vi "Dashboard Main.vi"() -> ()   [LabVIEW 2013]
uses:
  <vilib>/event_ctls.llb/eventvkey.ctl
  <vilib>/Rock Robotics/WPI/Dashboard/WPI_DashboardLogging Global.vi
  <vilib>/Utility/config.llb/Write Key (String).vi
  <vilib>/Utility/config.llb/Write Key (I32).vi
  <vilib>/Utility/config.llb/NI_LVConfig.lvlib
panel:
  out "code":string
  out "Image Message":string="Timeout in Camera Communications"
  in  "Rec Mode":enum32{"Stop", "Record", "Playback"}(radio)
  in  "Dashboard Tab":T1(tab)
  in  "Camera Settings":T2={"Frame Rate"=30, "Compression"=30, "Size"=1} {"Frame Rate" scale=1.0..30.0; "Size" items=["640x480", "320x240", "160x120"]}
  out "MotorSliders R":cluster{"MotorSlide1":dbl, "MotorSlide2":dbl} {"MotorSlide2" scale=-1.0..1.0 scale format="%#_2e"; "MotorSlide1" scale=-1.0..1.0 scale format="%#_2e"}
  out "MotorChart R":cluster{"Numeric":dbl, "Numeric":dbl}(graph)
  out "MotorSliders L":T3 {"MotorSlide4 2" scale=0.0..14.0 scale format="%#_2e"; "MotorSlide2" scale=-1.0..1.0 scale format="%#_2e"; "MotorSlide1" scale=-1.0..1.0 scale format="%#_2e"}
  out "MotorChart L":T4(graph)
  out "JS1 Z":dbl(slide) scale=-1.0..1.0 scale format="%#_2e"
  out "Joystick 1":cluster{"X":dbl, "Y":dbl}[](graph)
  out "JS Buttons 1":T5
  out "JS2 Z":dbl(slide) scale=-1.0..1.0 scale format="%#_2e"
  out "Joystick 2":cluster{"X":dbl, "Y":dbl}[](graph)
  out "JS Buttons 2":T5
  out "Mode":T6(ring)=enum."Auto Disabled"
  out "Camera IP":string
  in  "DB Camera Config":bool
  out "fps":dbl format="%#.1g"
  out "Mbps":dbl format="%#.1g"
  out "Mbps 2":bool
  out "LED 1":bool
  in  "loadCode":bool
  in  "pick auto":string
  out "left":dbl
  out "right":dbl
  out "Waveform Chart":dbl[][](graph)
  in  "Checkbox 2":bool
  in  "Checkbox 1":bool
  in  "Test Slider":dbl(slide) scale=0.0..100.0 scale format="%#_3g"
  in  "On/Off":bool caption="Solenoid"
  in  "Test Name":u16(ring) items=["Select the test to run...", "Example Test", "-------------------------------", "List of tests is built in robot code.", "Replace with your own automated tests."]
  in  "Test Tree":string(tree)
  in  "Motor":cluster{"Value":dbl, "Enable":bool} {"Value" scale=-1.0..1.0 scale format="%#_3g"}
  out "Progress":T7 {"Test Progress" scale=0.0..100.0}
  in  "Rev/Fwd":cluster{"Forward":bool, "Reverse":bool}
  in  "Test Ring":u16(ring) items=["Auto", "Fixed indoor", "Fixed outdoor 1", "Fixed outdoor 2", "Fixed fluorescent 1", "Fixed fluorescent 2", "Hold current"]
  in  "Listbox":i32(listbox)
  out "Tree":string(tree)
  out "Camera Image":T8(plugin-control)
  in  "Enable":bool
  # "Left"
  # "Front"
  # "Right"
  # "Battery"
  # "This tab is a great place for autonomous settings and validation.\nCustomize by placing controls and indicators here and name to\nmatch Dashboard Variables on robot."
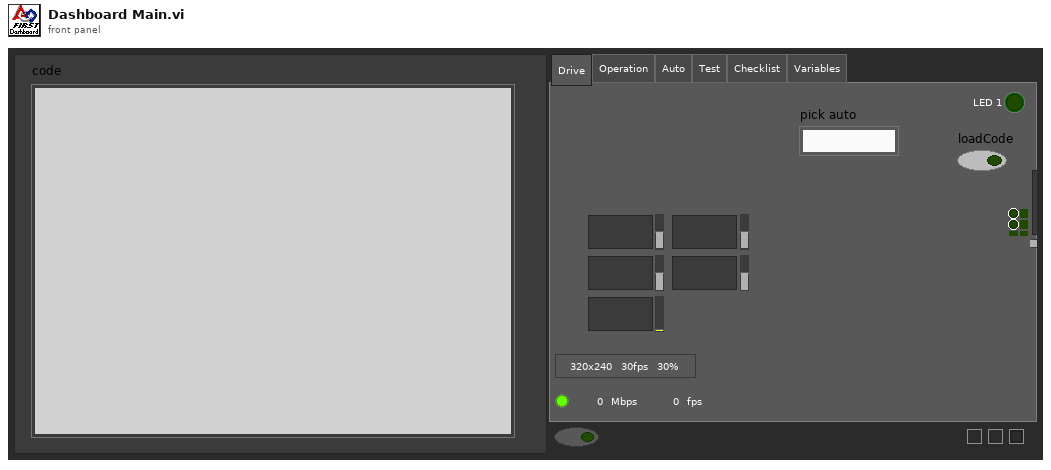
[diagram p1: front panel]
types:
  T1 = enum32{"Drive", "Operation", "Auto", "Test", "Checklist", "Variables"}
  T2 = cluster{"Frame Rate":i32, "Compression":i32, "Size":u16}
  T3 = cluster{"MotorSlide1":dbl, "MotorSlide2":dbl, "MotorSlide4 2":dbl}
  T4 = cluster{"Numeric":dbl, "Numeric":dbl, "Battery":sgl}
  T5 = cluster{bool, bool, bool, bool, bool, bool, bool, bool, bool, bool, bool, bool}
  T6 = enum8{"Tele-Op Disabled", "Tele-Op Enabled", "Auto Disabled", "Auto Enabled", "Test Disabled", "Test Enabled", ""}
  T7 = cluster{"Test Progress":u8, "Test Progress Text":string}
  T8 = typedef "IMAQ Image.ctl" = refnum<image>
  T9 = typedef "Image Type" = u32
  T10 = cluster{"Digital Inputs":bool[], "Digital Outputs":bool[]}
  T11 = cluster{"Competition mode":bool, "Robot Link":bool, "Autonomous":bool, "Enabled":bool, "E-Stop":bool, "Simulated":bool, "TestMode":bool, "Docked Window":bool}
  T12 = cluster{"Boolean Array[0]":bool, "Boolean Array[1]":bool, "Boolean Array[2]":bool, "Boolean Array[3]":bool, "Boolean Array[4]":bool, "Boolean Array[5]":bool, "Boolean Array[6]":bool, "Boolean Array[7]":bool, "Boolean Array[8]":bool, "Boolean Array[9]":bool, "Boolean Array[10]":bool, "Boolean Array[11]":bool}
  T13 = typedef "NI_LVConfig.lvlib/Config Data RefNum.ctl" = refnum<k1>
  T14 = typedef "eventvkey.ctl" = enum16{"ASCII", "Enter", "Return", "Shift", "Ctrl", "Alt", "Cmd", "Opt", "Caps", "NumLock", "Clear", "Break", "Up", "Down", "Left", "Right", "Insert", "Delete", "Home", "End", "PageUp", "PageDown", "Escape", "Help", "Pause", "ScrollLock", "F1", "F2", "F3", "F4", "F5", "F6", "F7", "F8", "F9", "F10", "F11", "F12", "F13", "F14", "F15", "F16", "F17", "F18", "F19", "F20", "F21", "F22", "F23", "F24", "Play", "VolumeUp", "VolumeDown", "Mute", "Two Byte Char"}
  T15 = cluster{"Image Size":bool, "Image Type":bool, "Pixel Value":bool, "ROI Information":bool, "Zoom Factor":bool}
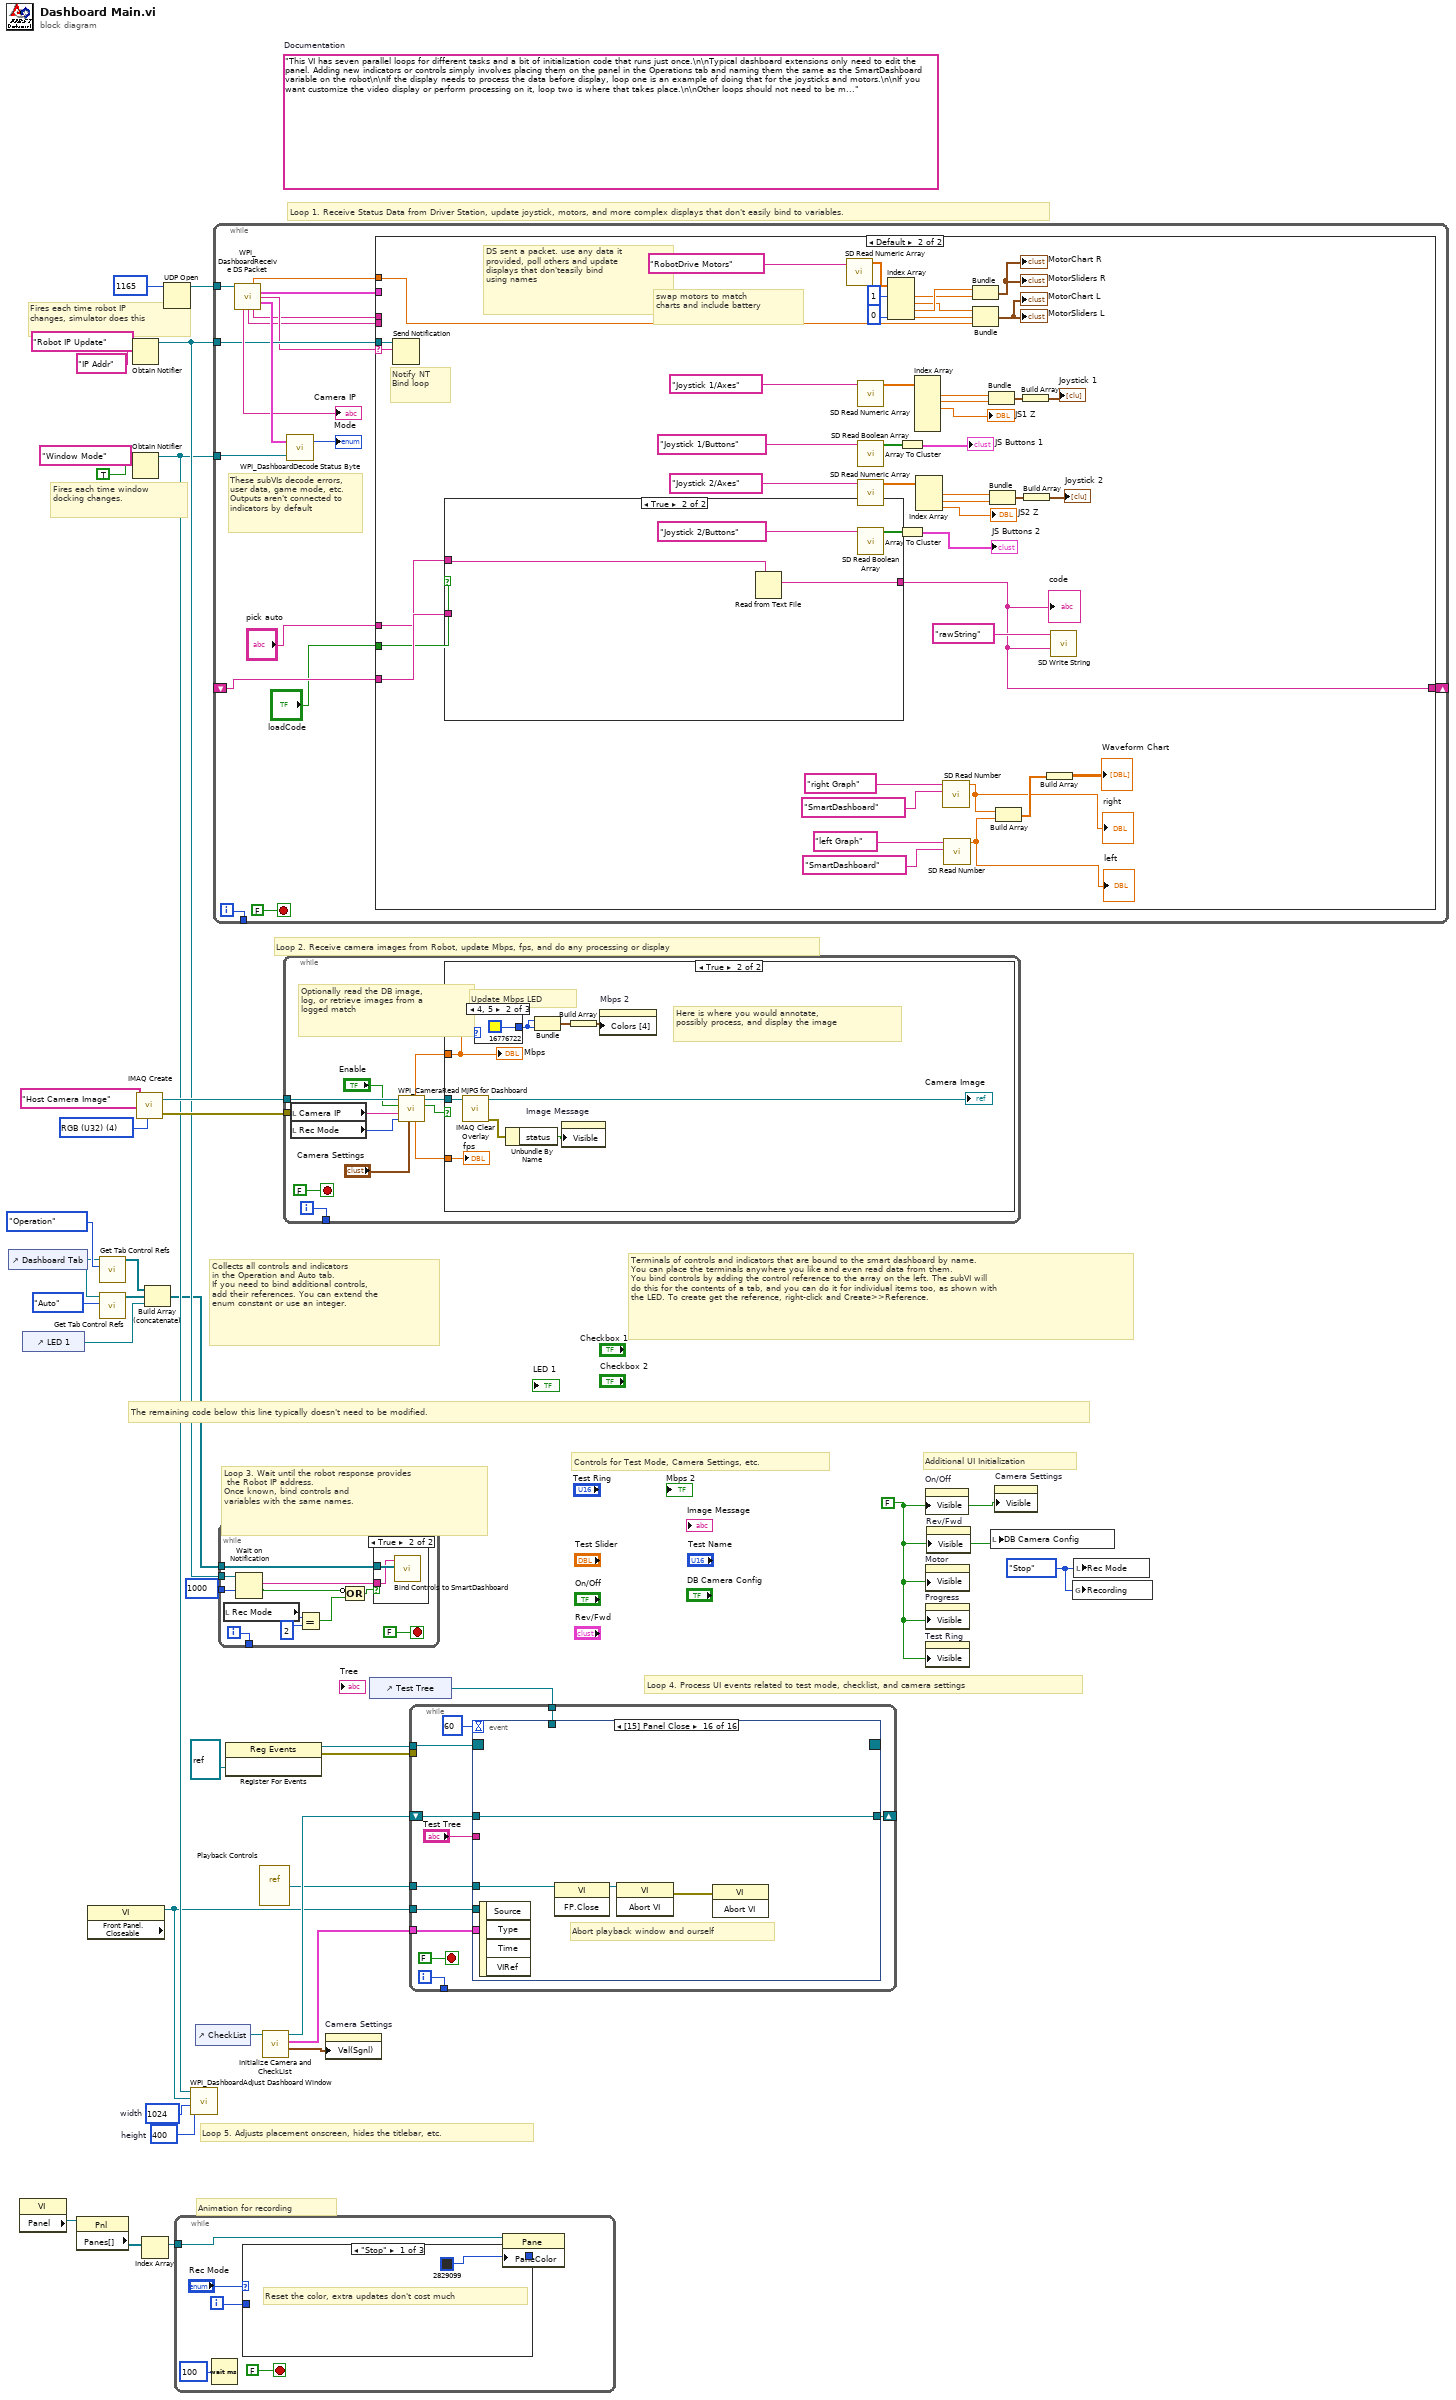
[diagram p0: block diagram]
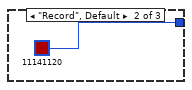
[diagram p2: hidden frame]
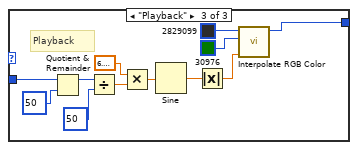
[diagram p3: hidden frame]
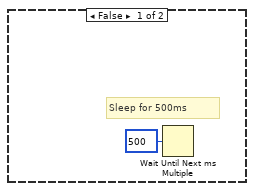
[diagram p5: hidden frame]
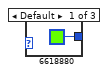
[diagram p6: hidden frame]
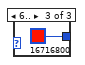
[diagram p7: hidden frame]
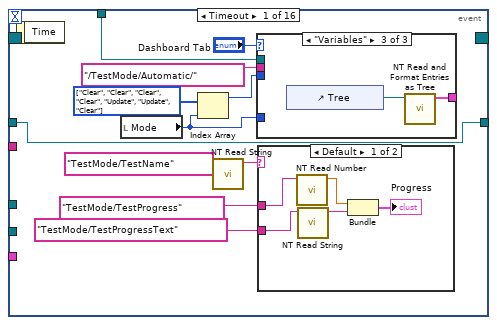
[diagram p8: hidden frame]
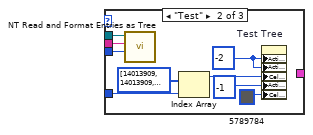
[diagram p10: hidden frame]
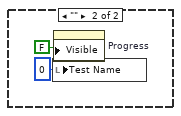
[diagram p11: hidden frame]
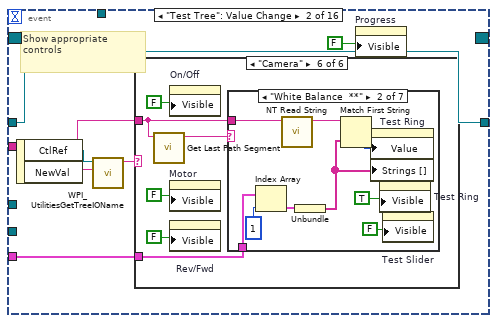
[diagram p12: hidden frame]
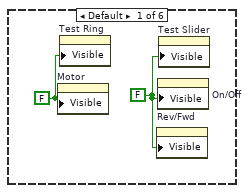
[diagram p13: hidden frame]
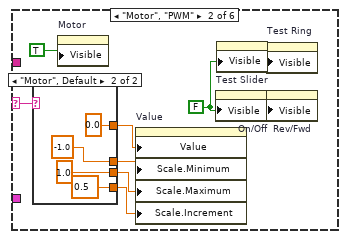
[diagram p14: hidden frame]
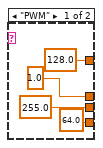
[diagram p15: hidden frame]
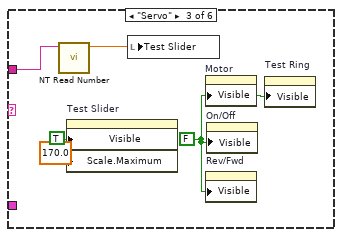
[diagram p16: hidden frame]
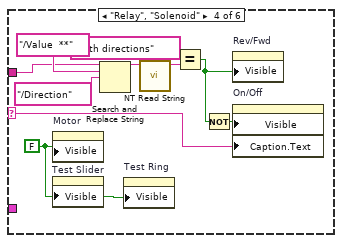
[diagram p17: hidden frame]
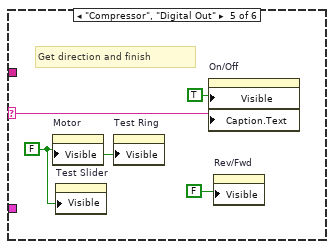
[diagram p18: hidden frame]
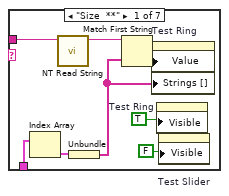
[diagram p19: hidden frame]
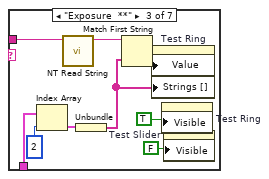
[diagram p20: hidden frame]
diagram:
  w8 = enum32{"Stop", "Record", "Playback"}."Stop" ("Rec Mode")
  w11 = 400  # height
  w12 = 1024  # width
  w25 = FALSE ("Visible")
  (unwired) "This VI has seven parallel loops for different tasks and a bit of initialization code that runs just once.\n\nTypical dashboard extensions only need to edit the panel. Adding new indicators or controls simply involves placing them on the panel in the Operations tab and naming them the same as the SmartDashboard variable on the robot\n\nIf the display needs to process the data before display, loop one is an example of doing that for the joysticks and motors.\n\nIf you want customize the video display or perform processing on it, loop two is where that takes place.\n\nOther loops should not need to be modified. They are pretty standard, and document the task they perform."  # Documentation
  w35 = T9 4 items=["Grayscale (U8)", "Grayscale (I16)", "Grayscale (SGL)", "Complex (CSG)", "RGB (U32)", "HSL (U32)", "RGB (U64)"] ("Image Type")
  # "Controls for Test Mode, Camera Settings, etc."
  # "Additional UI Initialization"
  # "Animation for recording"
  # "Fires each time robot IP\nchanges, simulator does this"
  # "Fires each time window\ndocking changes."
  # "Collects all controls and indicators\nin the Operation and Auto tab.\nIf you need to bind additional controls,\nadd their references. You can extend the\nenum constant or use an integer."
  # "The remaining code below this line typically doesn't need to be modified."
  # "Loop 4. Process UI events related to test mode, checklist, and camera settings"
  # "Terminals of controls and indicators that are bound to the smart dashboard by name.\nYou can place the terminals anywhere you like and even read data from them.\nYou bind controls by adding the control reference to the array on the left. The subVI will\ndo this for the contents of a tab, and you can do it for individual items too, as shown with\nthe LED. To create get the reference, right-click and Create>>Reference."
  # "Loop 3. Wait until the robot response provides\n the Robot IP address.\nOnce known, bind controls and\nvariables with the same names."
  # "Loop 5. Adjusts placement onscreen, hides the titlebar, etc."
  # "Loop 1. Receive Status Data from Driver Station, update joystick, motors, and more complex displays that don't easily bind to variables."
  # "Loop 2. Receive camera images from Robot, update Mbps, fps, and do any processing or display"
  n1 = control-ref of="Dashboard Tab"() -> (w6:refnum<vi>)
  n2 = property class="VI"() -> ("Panel"=w19:refnum<vi>)  [unwired: 2 in, 2 out]
  n3 = control-ref of="LED 1"() -> (w1:refnum<vi>)
  n4 = property class="Pnl"(reference=w19) -> ("Panes[]"=w20:refnum<vi>[])  [unwired: 1 in, 2 out]
  n5 = property class="VI" props=["Front Panel.Closeable"]() -> (reference out=w7:refnum<vi>)  [unwired: 2 in, 2 out]
  n6 = call <vilib>:"Get Tab Control Refs.vi"("Page Index"=T1."Operation" ("Dashboard Tab"), "TabControl in"=w6) -> ("ControlsOnPage"=w4:refnum<vi>[])  [unwired: 9 in]
  n7 = call <vilib>:"Get Tab Control Refs.vi"("Page Index"=T1."Auto" ("Dashboard Tab"), "TabControl in"=w6) -> ("ControlsOnPage"=w5:refnum<vi>[])  [unwired: 9 in]
  n8 = Obtain Notifier(name (unnamed)="Robot IP Update", notification data type="IP Addr" ("name (unnamed)")) -> (notifier out=w29:refnum<notifier>)  [unwired: 2 in, 2 out]
  n9 = Obtain Notifier(name (unnamed)="Window Mode", notification data type=TRUE) -> (notifier out=w10:refnum<notifier>)  [unwired: 2 in, 2 out]
  n10 = call "IMAQ Create"("Image Name"="Host Camera Image", "Image Type"=w35) -> ("New Image"=w33:T8, "error out"=w32:errorcluster)  [unwired: 2 in, 1 out]
  n11 = Index Array(array=w20) -> (element=w18:refnum<vi>)  [unwired: 1 in]
  n12 = Build Array (concatenate)(w4, w5, w1) -> (w3:refnum<vi>[])
  n13 = UDP Open(11:u16 1165 ("port")) -> (port=w36:refnum<k16>)  [unwired: 2 in, 4 out]
  n14 = while {
    tunnel: w18 -> [w40]
    i -> [w43]
    stop <- FALSE stop-if-true
    n15 = Wait (ms)(milliseconds to wait=u32 100) -> ()  [unwired: 1 out]
    n16 = case shown="\"Stop\"" "Rec Mode" {
      tunnel: w43 -> [_ _ w57]
      tunnel: [u32 2829099 ("Base Color") u32 11141120 ("Target Color") w46] -> w39
      frame "Stop" {
        # "Reset the color, extra updates don't cost much"
      }
      frame "Record", Default {
      }
      frame "Playback" {
        # "Playback"
        n17 = Quotient & Remainder(x=w57, y=u32 50 ("milliseconds to wait")) -> (x-y*floor(x/y)=w53:u32)  [unwired: 1 out]
        n18 = Divide(x=w53, y=u32 50 ("milliseconds to wait")) -> (x/y=w50:dbl)
        n19 = Multiply(x=6.283185307179586, y=w50) -> (x*y=w55:dbl)
        n20 = Sine(x=w55) -> (sin(x)=w54:dbl)
        n21 = Absolute Value(x=w54) -> (abs(x)=w47:dbl)
        n22 = call "Interpolate RGB Color.vi"("Proportion"=w47, "Target Color"=u32 30976, "Base Color"=u32 2829099) -> ("Result Color"=w46:u32)  [unwired: 8 in]
      }
    }
    n23 = property class="Pane"(reference=w40, "PaneColor"=w39) -> ()  [unwired: 1 in, 2 out]
  }
  n24 = call <vilib>:"WPI_DashboardAdjust Dashboard Window.vi"("height"=w11, "width"=w12, "reference in"=w7, "Notifier in"=w10) -> ()  [unwired: 8 in]
  n25 = control-ref of="CheckList"() -> (w9:refnum<vi>)
  n26 = while {
    tunnel: w36 -> [w73]
    tunnel: w29 -> [w68]
    tunnel: w10 -> [w72]
    tunnel: [w69] -> _
    shift-right: [w60] -> _
    shift-left: _ -> [w61]
    i -> [w69]
    stop <- FALSE stop-if-true
    # "These subVIs decode errors, user data, game mode, etc.\nOutputs aren't connected to indicators by default"
    n27 = call <vilib>:"WPI_DashboardReceive DS Packet.vi"("Recv Socket"=w73) -> ("Battery"=w63:sgl, "Driver Station"=w64:T10, "Robot IP Address"=w67:string, "Status"=w74:T11, "Camera IP Address"=→"Camera IP":string, "Low Priority User Data"=w66:string, "High Priority User Data"=w65:string)  [unwired: 1 in, 7 out]
    n28 = call <vilib>:"WPI_DashboardDecode Status Byte.vi"("Window Mode Notifier"=w72, "Status"=w74) -> ("Mode"=→"Mode":T6)  [unwired: 1 out]
    n29 = case shown="Default" w67 {
      selector: w67 -> [_ w99]
      tunnel: w68 -> [_ w100]
      tunnel: w66 -> [_ _]
      tunnel: w65 -> [_ _]
      tunnel: w64 -> [_ _]
      tunnel: w63 -> [_ w98]
      tunnel: w61 -> [w75 w87]
      tunnel: [w75 w76] -> w60
      tunnel: "pick auto" -> [_ w86]
      tunnel: "loadCode" -> [_ w85]
      frame "0.0.0.0" {
        # "DS not sending packets, or no robot exists yet.\nDon't poll the variables"
      }
      frame Default {
        # "Notify NT\nBind loop"
        # "DS sent a packet. use any data it\nprovided, poll others and update\ndisplays that don'teasily bind\nusing names"
        # "swap motors to match\ncharts and include battery"
        n30 = Send Notification(notification=w99, notifier=w100) -> ()  [unwired: 1 in, 2 out]
        n31 = case shown="True" w85 {
          tunnel: [w122 w124] -> w76
          tunnel: w87 -> [w122 _]
          tunnel: w86 -> [_ w123]
          frame False {
          }
          frame True {
            n32 = Read from Text File(prompt (Open existing file)=w123) -> (text=w124:string)  [unwired: 3 in, 3 out]
          }
        }
        "code" <- w76
        n33 = call <vilib>:"SD Read Numeric Array.vi"("Name"="RobotDrive Motors") -> ("Numeric Array"=w97:dbl[])  [unwired: 8 in, 2 out]
        n34 = call <vilib>:"SD Read Numeric Array.vi"("Name"="Joystick 1/Axes") -> ("Numeric Array"=w116:dbl[])  [unwired: 8 in, 2 out]
        n35 = call <vilib>:"SD Read Boolean Array.vi"("Name"="Joystick 1/Buttons") -> ("Boolean Array"=w118:bool[])  [unwired: 8 in, 2 out]
        n36 = call <vilib>:"SD Read Numeric Array.vi"("Name"="Joystick 2/Axes") -> ("Numeric Array"=w110:dbl[])  [unwired: 8 in, 2 out]
        n37 = call <vilib>:"SD Read Boolean Array.vi"("Name"="Joystick 2/Buttons") -> ("Boolean Array"=w109:bool[])  [unwired: 8 in, 2 out]
        n38 = Index Array(array=w97, index #1=1, index #4=0) -> (element #1=w93:dbl, element #2=w92:dbl, element #3=w94:dbl, element #4=w89:dbl)  [unwired: 2 in]
        n39 = Array To Cluster(array=w118) -> (cluster=→"JS Buttons 1":T12)
        n40 = Array To Cluster(array=w109) -> (cluster=→"JS Buttons 2":T12)
        n41 = Index Array(array=w116) -> (element #1=w113:dbl, element #2=w114:dbl, element #3=→"JS1 Z":dbl)  [unwired: 6 in, 3 out]
        n42 = Index Array(array=w110) -> (element #1=w105:dbl, element #2=w104:dbl, element #3=→"JS2 Z":dbl)  [unwired: 3 in]
        n43 = call <vilib>:"SD Read Number.vi"("Table Prefix"="SmartDashboard", "Name"="right Graph") -> ("Numeric"=w78:dbl)  [unwired: 7 in, 2 out]
        "right" <- w78
        n44 = call <vilib>:"SD Read Number.vi"("Table Prefix"="SmartDashboard", "Name"="left Graph") -> ("Numeric"=w77:dbl)  [unwired: 7 in, 2 out]
        "left" <- w77
        n45 = Bundle("Numeric"=w94, "Numeric"=w93) -> (→"MotorChart R" →"MotorSliders R":cluster{"Numeric":dbl, "Numeric":dbl})  [unwired: 1 in]
        n46 = Bundle("Numeric"=w92, "Numeric"=w89, "Battery"=w98) -> (→"MotorChart L" →"MotorSliders L":T4)  [unwired: 1 in]
        n47 = Bundle("Numeric"=w113, "Numeric"=w114) -> (w112:cluster{"Numeric":dbl, "Numeric":dbl})  [unwired: 1 in]
        n48 = Bundle("Numeric"=w105, "Numeric"=w104) -> (w106:cluster{"Numeric":dbl, "Numeric":dbl})  [unwired: 1 in]
        n49 = Build Array(w78, w77) -> (w80:dbl[])
        n50 = Build Array(w112) -> (→"Joystick 1":cluster{"Numeric":dbl, "Numeric":dbl}[])
        n51 = Build Array(w106) -> (→"Joystick 2":cluster{"Numeric":dbl, "Numeric":dbl}[])
        n52 = Build Array(w80) -> (→"Waveform Chart":dbl[][])
        n53 = call <vilib>:"SD Write String.vi"("String"=w76, "Name"="rawString") -> ()  [unwired: 8 in, 2 out]
      }
    }
  }
  n54 = while {
    tunnel: w3 -> [w135]
    tunnel: w29 -> [w134]
    tunnel: [w132] -> _
    tunnel: u32 1000 ("milliseconds to wait") -> [w131]
    i -> [w132]
    stop <- FALSE stop-if-true
    n55 = local read "Rec Mode"() -> (w127:enum32{"Stop", "Record", "Playback"})
    n56 = Wait on Notification(notifier=w134, timeout in ms (-1)=w131) -> (notification=w133:string, timed out?=w129:bool)  [unwired: 2 in, 2 out]
    n57 = Equal?(x=w127, y=u16 2 ("Rec Mode")) -> (x = y?=w128:bool)
    n58 = Compound Arithmetic op=OR(invert w129, w128) -> (w130:bool)
    n59 = case shown="True" w130 {
      tunnel: w135 -> [_ w137]
      tunnel: w133 -> [_ w136]
      frame False {
      }
      frame True {
        n60 = call <vilib>:"Bind Controls to SmartDashboard.vi"("Bound Control Refs"=w137, "Server IP Address"=w136) -> ()  [unwired: 10 in]
      }
    }
  }
  n61 = register-events(refnum<vi> refnum) -> (reference out=w16:refnum<event-registration>, error out=w15:errorcluster)  [unwired: 2 in]
  n62 = vi-ref "Playback Controls.vi"() -> (w17:refnum<vi>)
  n63 = call "Initialize Camera and CheckList.vi"("ListBox in"=w9) -> ("Cluster"=w23:cluster{"value":i32, "value":i32, "index":i32}, "Array"=w24:cluster{string[]}[], "File Refnum"=w22:T13)  [unwired: 8 in]
  n64 = while {
    tunnel: w33 -> [w147]
    tunnel: w32 -> [_]
    tunnel: [w148] -> _
    i -> [w148]
    stop <- FALSE stop-if-true
    # "Optionally read the DB image,\nlog, or retrieve images from a\nlogged match"
    n65 = local read "Camera IP"() -> (w140:string)
    n66 = local read "Rec Mode"() -> (w139:enum32{"Stop", "Record", "Playback"})
    n67 = call <vilib>:"WPI_CameraRead MJPG for Dashboard.vi"("Camera Settings"="Camera Settings", "Rec Mode"=w139, "Camera IP"=w140, "Enable"="Enable", "Refnum in"=w147) -> ("Active"=w144:bool, "Refnum out"=w146:T8, "FPS"=w143:dbl, "Bandwidth (Mbps)"=w142:dbl)  [unwired: 3 in]
    n68 = case shown="True" w144 {
      tunnel: w146 -> [_ w153]
      tunnel: w142 -> [_ w152]
      tunnel: w143 -> [_ w150]
      frame False {
        # "Sleep for 500ms"
        n69 = Wait Until Next ms Multiple(millisecond multiple=u32 500) -> ()  [unwired: 1 out]
      }
      frame True {
        # "Here is where you would annotate,\npossibly process, and display the image"
        # "Update Mbps LED"
        n70 = call "IMAQ Clear Overlay"("Image"=w153) -> ("error out"=w157:errorcluster, "Image Out"=→"Camera Image":T8)  [unwired: 2 in, 7 out]
        n71 = case shown="4, 5" w152 {
          tunnel: [u32 6618880 ("Color Box") u32 16776722 ("Color Box") u32 16716800 ("Color Box")] -> w154
          frame Default {
          }
          frame 4, 5 {
          }
          frame 6.. {
          }
        }
        n72 = Unbundle By Name(w157) -> ("status"=w158:bool)
        n73 = Bundle("Color Box"=w154, "Color Box"=w154) -> (w156:cluster{"Color Box":u32, "Color Box":u32})  [unwired: 1 out]
        n74 = property on="Image Message" class="Str"("Visible"=w158) -> ()  [unwired: 2 in, 2 out]
        n75 = Build Array(w156) -> (w155:cluster{"Color Box":u32, "Color Box":u32}[])
        n76 = property on="Mbps 2" class="Bool (strict)"("Colors [4]"=w155) -> ()  [unwired: 2 in, 2 out]
        "Mbps" <- w152
        "fps" <- w150
      }
    }
  }
  n77 = property on="Camera Settings" class="Clust (strict)"("Val(Sgnl)"=w23) -> ()  [unwired: 2 in, 2 out]
  n78 = control-ref of="Test Tree"() -> (w21:refnum<vi>)
  n79 = while {
    tunnel: w24 -> [w170]
    shift-right: [w169] -> _
    shift-left: w22 -> [w168]
    tunnel: [w167] -> _
    tunnel: w21 -> [w166]
    tunnel: w17 -> [w165]
    tunnel: w16 -> [w164]
    tunnel: w15 -> [_]
    tunnel: w7 -> [w163]
    i -> [w167]
    stop <- FALSE stop-if-true
    n80 = event shown="[15] Panel Close" {
      selector: w164 -> [_ _ _ _ _ _ _ _ _ _ _ _ _ _ _ _]
      dyn-events: [_ _ _ _ _ _ _ _ _ _ _ _ _ w407 _ _] -> _
      timeout: u32 60 ("milliseconds to wait") -> [_ _ _ _ _ _ _ _ _ _ _ _ _ _ _ _]
      tunnel: w166 -> [w179 _ _ _ _ _ _ _ _ _ _ _ _ _ _ _]
      tunnel: "Test Tree" -> [_ _ _ _ _ _ _ _ w376 w384 w386 w390 w398 _ _ _]
      tunnel: w170 -> [_ w203 _ _ _ _ w340 w370 _ _ _ _ _ _ _ _]
      tunnel: [w173 w202 w301 w306 w314 w326 w339 w363 w375 w382 w385 w389 w397 w409 w423 w424] -> w169
      tunnel: w168 -> [w173 w202 w301 w306 w314 w326 w338 w363 w375 w382 w385 w389 w397 w409 w423 w424]
      tunnel: w165 -> [_ _ _ _ _ _ _ _ _ _ _ _ _ w410 _ w427]
      tunnel: w163 -> [_ _ _ _ _ _ _ _ _ _ _ _ _ w405 _ _]
      event Timeout {
        w178 = enum16{"Update", "Clear"}[] [enum."Clear", enum."Clear", enum."Clear", enum."Clear", enum."Update", enum."Update", enum."Clear"] items=["Update", "Clear"]
        n81 = event-data() -> ()  [unwired: 1 in, 1 out]
        n82 = local read "Mode"() -> (w176:T6)
        n83 = Index Array(array=w178, index=w176) -> (element=w177:enum16{"Update", "Clear"})
        n84 = call <vilib>:"NT Read String.vi"("Name"="TestMode/TestName") -> ("String"=w182:string)  [unwired: 9 in, 1 out]
        n85 = case shown="\"Variables\"" "Dashboard Tab" {
          tunnel: w179 -> [_ w192 _]
          tunnel: "/TestMode/Automatic/" ("Name Pattern") -> [_ w191 _]
          tunnel: w177 -> [_ w190 _]
          tunnel: w176 -> [_ w188 _]
          tunnel: [_ _ w194] -> _
          frame "Operation", Default {
          }
          frame "Test" {
            w187 = -2 ("Active Item:Row Number")
            n86 = call <vilib>:"NT Read and Format Entries as Tree.vi"("Operation"=w190, "Name Pattern"=w191, "Tree Refnum"=w192) -> ()  [unwired: 7 in, 2 out]
            n87 = Index Array(array=u32[] [14013909, 14013909, 14013909, 14013909, 14013909, 16777215, 14013909], index=w188) -> (element=w186:u32)
            n88 = property on="Test Tree" class="Tree (strict)"("Active Item Row Number"=w187, "ActiveColNum"=w187, "CellBG"=w186, "Active Item Row Number"=-1 ("Active Item:Row Number"), "CellBG"=u32 5789784 ("Color Box")) -> ()  [unwired: 2 in, 2 out]
          }
          frame "Variables" {
            n89 = control-ref of="Tree"() -> (w193:refnum<vi>)
            n90 = call <vilib>:"NT Read and Format Entries as Tree.vi"("Tree Refnum"=w193) -> ("Formatted Strings"=w194:cluster{"Name":string, "Value":string}[])  [unwired: 9 in, 1 out]
          }
        }
        n91 = case shown="Default" w182 {
          tunnel: "TestMode/TestProgress" ("Name") -> [w196 _]
          tunnel: "TestMode/TestProgressText" ("Name") -> [w195 _]
          frame Default {
            n92 = call <vilib>:"NT Read Number.vi"("Name"=w196) -> ("Numeric"=w197:dbl)  [unwired: 9 in, 1 out]
            n93 = call <vilib>:"NT Read String.vi"("Name"=w195) -> ("String"=w198:string)  [unwired: 9 in, 1 out]
            n94 = Bundle("Numeric"=w197, "String"=w198) -> (→"Progress":cluster{"Numeric":dbl, "String":string})  [unwired: 1 in]
          }
          frame "" {
            n95 = local write "Test Name"(u16 0) -> ()
            n96 = property on="Progress" class="Clust (strict)"("Visible"=FALSE) -> ()  [unwired: 2 in, 2 out]
          }
        }
      }
      event "Test Tree": Value Change {
        # "Show appropriate\ncontrols"
        n97 = event-data() -> ("CtlRef"=w206:refnum<vi>, "NewVal"=w204:string)  [unwired: 1 in]
        n98 = call <vilib>:"WPI_UtilitiesGetTreeIOName.vi"("NewVal"=w204, "TreeControl in"=w206) -> ("I/O Name"=w207:string)  [unwired: 9 in]
        n99 = case shown="\"Camera\"" w207 {
          selector: w207 -> [_ w214 _ w232 w241 _]
          tunnel: w204 -> [_ _ w229 w231 _ w248]
          tunnel: w203 -> [_ _ _ _ _ w247]
          frame Default {
            w209 = FALSE ("Visible")
            w208 = FALSE ("Visible")
            n100 = property on="Motor" class="Clust (strict)"("Visible"=w208) -> ()  [unwired: 2 in, 2 out]
            n101 = property on="Test Ring" class="Ring (strict)"("Visible"=w208) -> ()  [unwired: 2 in, 2 out]
            n102 = property on="Rev/Fwd" class="Clust (strict)"("Visible"=w209) -> ()  [unwired: 2 in, 2 out]
            n103 = property on="On/Off" class="Bool (strict)"("Visible"=w209) -> ()  [unwired: 2 in, 2 out]
            n104 = property on="Test Slider" class="Slide (strict)"("Visible"=w209) -> ()  [unwired: 2 in, 2 out]
          }
          frame "Motor", "PWM" {
            w215 = FALSE ("Visible")
            n105 = case shown="\"Motor\", Default" w214 {
              tunnel: [1.0 ("Value") -1.0 ("Value")] -> w213
              tunnel: [255.0 ("Value") 1.0 ("Value")] -> w212
              tunnel: [128.0 ("Value") 0.0 ("Value")] -> w211
              tunnel: [64.0 ("Value") 0.5 ("Value")] -> w210
              frame "PWM" {
              }
              frame "Motor", Default {
              }
            }
            n106 = property on="Motor" class="Clust (strict)"("Visible"=TRUE) -> ()  [unwired: 2 in, 2 out]
            n107 = property on="Value" class="Slide (strict)"("Value"=w211, "Scale.Minimum"=w213, "Scale.Maximum"=w212, "Scale.Increment"=w210) -> ()  [unwired: 2 in, 2 out]
            n108 = property on="On/Off" class="Bool (strict)"("Visible"=w215) -> ()  [unwired: 2 in, 2 out]
            n109 = property on="Test Slider" class="Slide (strict)"("Visible"=w215) -> ()  [unwired: 2 in, 2 out]
            n110 = property on="Test Ring" class="Ring (strict)"("Visible"=w215) -> ()  [unwired: 2 in, 2 out]
            n111 = property on="Rev/Fwd" class="Clust (strict)"("Visible"=w215) -> ()  [unwired: 2 in, 2 out]
          }
          frame "Servo" {
            w227 = FALSE ("Visible")
            n112 = call <vilib>:"NT Read Number.vi"("Name"=w229) -> ("Numeric"=w228:dbl)  [unwired: 9 in, 1 out]
            n113 = property on="Test Slider" class="Slide (strict)"("Visible"=TRUE, "Scale.Maximum"=170.0 ("Scale.Range:Maximum")) -> ()  [unwired: 2 in, 2 out]
            n114 = local write "Test Slider"(w228) -> ()
            n115 = property on="Motor" class="Clust (strict)"("Visible"=w227) -> ()  [unwired: 2 in, 2 out]
            n116 = property on="Rev/Fwd" class="Clust (strict)"("Visible"=w227) -> ()  [unwired: 2 in, 2 out]
            n117 = property on="On/Off" class="Bool (strict)"("Visible"=w227) -> ()  [unwired: 2 in, 2 out]
            n118 = property on="Test Ring" class="Ring (strict)"("Visible"=w227) -> ()  [unwired: 2 in, 2 out]
          }
          frame "Relay", "Solenoid" {
            w230 = FALSE ("Visible")
            n119 = property on="Motor" class="Clust (strict)"("Visible"=w230) -> ()  [unwired: 2 in, 2 out]
            n120 = property on="Test Slider" class="Slide (strict)"("Visible"=w230) -> ()  [unwired: 2 in, 2 out]
            n121 = Search and Replace String(input string=w231, search string="/Value  **", replace string="/Direction") -> (result string=w237:string)  [unwired: 5 in, 3 out]
            n122 = property on="Test Ring" class="Ring (strict)"("Visible"=w230) -> ()  [unwired: 2 in, 2 out]
            n123 = call <vilib>:"NT Read String.vi"("Name"=w237) -> ("String"=w235:string)  [unwired: 9 in, 1 out]
            n124 = Equal?(x="Both directions", y=w235) -> (x = y?=w233:bool)
            n125 = Not(x=w233) -> (.not. x?=w234:bool)
            n126 = property on="Rev/Fwd" class="Clust (strict)"("Visible"=w233) -> ()  [unwired: 2 in, 2 out]
            n127 = property on="On/Off" class="Bool (strict)"("Visible"=w234, "Caption.Text"=w232) -> ()  [unwired: 2 in, 2 out]
          }
          frame "Compressor", "Digital Out" {
            w240 = FALSE ("Visible")
            # "Get direction and finish"
            n128 = property on="Motor" class="Clust (strict)"("Visible"=w240) -> ()  [unwired: 2 in, 2 out]
            n129 = property on="Test Slider" class="Slide (strict)"("Visible"=w240) -> ()  [unwired: 2 in, 2 out]
            n130 = property on="Test Ring" class="Ring (strict)"("Visible"=w240) -> ()  [unwired: 2 in, 2 out]
            n131 = property on="On/Off" class="Bool (strict)"("Visible"=TRUE, "Caption.Text"=w241) -> ()  [unwired: 2 in, 2 out]
            n132 = property on="Rev/Fwd" class="Clust (strict)"("Visible"=FALSE) -> ()  [unwired: 2 in, 2 out]
          }
          frame "Camera" {
            n133 = call <vilib>:"Get Last Path Segment.vi"("String in"=w248) -> ("String out"=w249:string)  [unwired: 10 in]
            n134 = property on="On/Off" class="Bool (strict)"("Visible"=FALSE) -> ()  [unwired: 2 in, 2 out]
            n135 = property on="Motor" class="Clust (strict)"("Visible"=FALSE) -> ()  [unwired: 2 in, 2 out]
            n136 = property on="Rev/Fwd" class="Clust (strict)"("Visible"=FALSE) -> ()  [unwired: 2 in, 2 out]
            n137 = case shown="\"White Balance  **\"" w249 {
              tunnel: w248 -> [w255 w264 w273 w282 w291 _ w297]
              tunnel: w247 -> [w253 w261 w270 w279 w288 _ _]
              frame "Size  **" {
                n138 = Index Array(array=w253) -> (element=w252:cluster{string[]})  [unwired: 1 in]
                n139 = call <vilib>:"NT Read String.vi"("Name"=w255) -> ("String"=w254:string)  [unwired: 9 in, 1 out]
                n140 = Unbundle(w252) -> (w250:string[])
                n141 = Match First String(2:w250, 3:w254) -> (0:w251:i32)  [unwired: 1 out]
                n142 = property on="Test Ring" class="Ring (strict)"("Value"=w251, "Strings []"=w250) -> ()  [unwired: 2 in, 2 out]
                n143 = property on="Test Ring" class="Ring (strict)"("Visible"=TRUE) -> ()  [unwired: 2 in, 2 out]
                n144 = property on="Test Slider" class="Slide (strict)"("Visible"=FALSE) -> ()  [unwired: 2 in, 2 out]
              }
              frame "White Balance  **" {
                n145 = Index Array(array=w261, index=1) -> (element=w262:cluster{string[]})
                n146 = call <vilib>:"NT Read String.vi"("Name"=w264) -> ("String"=w263:string)  [unwired: 9 in, 1 out]
                n147 = Unbundle(w262) -> (w259:string[])
                n148 = Match First String(2:w259, 3:w263) -> (0:w258:i32)  [unwired: 1 out]
                n149 = property on="Test Ring" class="Ring (strict)"("Value"=w258, "Strings []"=w259) -> ()  [unwired: 2 in, 2 out]
                n150 = property on="Test Ring" class="Ring (strict)"("Visible"=TRUE) -> ()  [unwired: 2 in, 2 out]
                n151 = property on="Test Slider" class="Slide (strict)"("Visible"=FALSE) -> ()  [unwired: 2 in, 2 out]
              }
              frame "Exposure  **" {
                n152 = Index Array(array=w270, index=2) -> (element=w271:cluster{string[]})
                n153 = call <vilib>:"NT Read String.vi"("Name"=w273) -> ("String"=w272:string)  [unwired: 9 in, 1 out]
                n154 = Unbundle(w271) -> (w267:string[])
                n155 = Match First String(2:w267, 3:w272) -> (0:w268:i32)  [unwired: 1 out]
                n156 = property on="Test Ring" class="Ring (strict)"("Value"=w268, "Strings []"=w267) -> ()  [unwired: 2 in, 2 out]
                n157 = property on="Test Ring" class="Ring (strict)"("Visible"=TRUE) -> ()  [unwired: 2 in, 2 out]
                n158 = property on="Test Slider" class="Slide (strict)"("Visible"=FALSE) -> ()  [unwired: 2 in, 2 out]
              }
              frame "Exposure Priority  **" {
                n159 = Index Array(array=w279, index=3) -> (element=w280:cluster{string[]})
                n160 = call <vilib>:"NT Read String.vi"("Name"=w282) -> ("String"=w281:string)  [unwired: 9 in, 1 out]
                n161 = Unbundle(w280) -> (w276:string[])
                n162 = Match First String(2:w276, 3:w281) -> (0:w277:i32)  [unwired: 1 out]
                n163 = property on="Test Ring" class="Ring (strict)"("Value"=w277, "Strings []"=w276) -> ()  [unwired: 2 in, 2 out]
                n164 = property on="Test Ring" class="Ring (strict)"("Visible"=TRUE) -> ()  [unwired: 2 in, 2 out]
                n165 = property on="Test Slider" class="Slide (strict)"("Visible"=FALSE) -> ()  [unwired: 2 in, 2 out]
              }
              frame "Color Enable  **" {
                n166 = Index Array(array=w288, index=4) -> (element=w289:cluster{string[]})
                n167 = call <vilib>:"NT Read String.vi"("Name"=w291) -> ("String"=w290:string)  [unwired: 9 in, 1 out]
                n168 = Unbundle(w289) -> (w285:string[])
                n169 = Match First String(2:w285, 3:w290) -> (0:w286:i32)  [unwired: 1 out]
                n170 = property on="Test Ring" class="Ring (strict)"("Value"=w286, "Strings []"=w285) -> ()  [unwired: 2 in, 2 out]
                n171 = property on="Test Ring" class="Ring (strict)"("Visible"=TRUE) -> ()  [unwired: 2 in, 2 out]
                n172 = property on="Test Slider" class="Slide (strict)"("Visible"=FALSE) -> ()  [unwired: 2 in, 2 out]
              }
              frame Default {
                n173 = property on="Test Ring" class="Ring (strict)"("Visible"=FALSE) -> ()  [unwired: 2 in, 2 out]
                n174 = property on="Test Slider" class="Slide (strict)"("Visible"=FALSE) -> ()  [unwired: 2 in, 2 out]
              }
              frame "Brightness  **", "Color Level  **", "Compression  **", "FPS  **", "Sharpness  **" {
                n175 = call <vilib>:"NT Read Number.vi"("Name"=w297) -> ("Numeric"=w296:dbl)  [unwired: 9 in, 1 out]
                n176 = local write "Test Slider"(w296) -> ()
                n177 = property on="Test Slider" class="Slide (strict)"("Visible"=TRUE, "Scale.Maximum"=100.0 ("Scale.Range:Maximum")) -> ()  [unwired: 2 in, 2 out]
                n178 = property on="Test Ring" class="Ring (strict)"("Visible"=FALSE) -> ()  [unwired: 2 in, 2 out]
              }
            }
          }
        }
        n179 = property on="Progress" class="Clust (strict)"("Visible"=FALSE) -> ()  [unwired: 2 in, 2 out]
      }
      event "Test Name": Mouse Enter {
        # "Populate the ring with the list of tests"
        n180 = event-data() -> ()  [unwired: 1 in, 1 out]
        n181 = call <vilib>:"NT Read String Array.vi"("Name"="TestMode/TestList") -> ("String Array"=w305:string[])  [unwired: 9 in, 1 out]
        n182 = Build Array (concatenate)("Select the test to run...", w305) -> (w304:string[])
        n183 = property on="Test Name" class="Ring (strict)"("Strings []"=w304) -> ()  [unwired: 2 in, 2 out]
      }
      event "Test Name": Value Change {
        w307 = FALSE ("Visible")
        # "Tell the robot the test name to run"
        n184 = event-data() -> ("NewVal"=w311:u16)  [unwired: 1 in]
        n185 = property on="Test Name" class="Ring (strict)"() -> ("Strings []"=w312:string[])  [unwired: 2 in, 2 out]
        n186 = local write "Progress"(T7 {"Test Progress"=0, "Test Progress Text"=""} ("Progress")) -> ()
        n187 = Index Array(array=w312, index=w311) -> (element=w310:string)
        n188 = call <vilib>:"NT Write String.vi"("String"=w310, "Name"="TestMode/TestName") -> ()  [unwired: 9 in, 1 out]
        n189 = property on="Progress" class="Clust (strict)"("Visible"=TRUE) -> ()  [unwired: 2 in, 2 out]
        n190 = property on="Motor" class="Clust (strict)"("Visible"=w307) -> ()  [unwired: 2 in, 2 out]
        n191 = property on="Test Slider" class="Slide (strict)"("Visible"=w307) -> ()  [unwired: 2 in, 2 out]
        n192 = property on="On/Off" class="Bool (strict)"("Visible"=w307) -> ()  [unwired: 2 in, 2 out]
        n193 = property on="Rev/Fwd" class="Clust (strict)"("Visible"=w307) -> ()  [unwired: 2 in, 2 out]
        n194 = property on="Test Ring" class="Ring (strict)"("Visible"=w307) -> ()  [unwired: 2 in, 2 out]
      }
      event "Listbox": Double Click {
        n195 = event-data() -> ("PlatMods.Shift"=w315:bool, "Row"=w317:i32)  [unwired: 1 in]
        n196 = case shown="True" w315 {
          tunnel: w317 -> [w321 _]
          tunnel: 1 -> [w320 _]
          frame False {
            n197 = property on="Listbox" class="LstBox (strict)"() -> ("Item Symbols"=w319:i32[])  [unwired: 2 in, 2 out]
            n198 = Replace Array Subset(array=w319, new element=w320, index=w321) -> (w318:i32[])
            n199 = property on="Listbox" class="LstBox (strict)"("Item Symbols"=w318) -> ()  [unwired: 2 in, 2 out]
          }
          frame True {
            w322 = 0 ("Top Row")
            n200 = property on="Listbox" class="LstBox (strict)"() -> ("Number of Rows"=w324:u32)  [unwired: 2 in, 2 out]
            n201 = Initialize Array(0, w324) -> (w323:i32[])
            n202 = property on="Listbox" class="LstBox (strict)"("Top Row"=w322, "Value"=w322, "Item Symbols"=w323) -> ()  [unwired: 2 in, 2 out]
          }
        }
      }
      event "Listbox": Key Down {
        n203 = event-data() -> ("VKey"=w328:T14)  [unwired: 1 in]
        n204 = case shown="\"Left\", \"Right\"" w328 {
          selector: w328 -> [w333 _]
          tunnel: eventvkey."Left" ("VKey") -> [w331 _]
          frame "Left", "Right" {
            n205 = Equal?(x=w331, y=w333) -> (x = y?=w332:bool)
            n206 = Select(t=0, s=w332, f=1) -> (s? t:f=w334:i32)
            n207 = property on="Listbox" class="LstBox (strict)"() -> ("Item Symbols"=w337:i32[])  [unwired: 2 in, 2 out]
            n208 = Replace Array Subset(array=w337, new element=w334, index="Listbox") -> (w336:i32[])
            n209 = property on="Listbox" class="LstBox (strict)"("Item Symbols"=w336) -> ()  [unwired: 2 in, 2 out]
          }
          frame Default {
          }
        }
      }
      event "DB Camera Config": Value Change {
        n210 = event-data() -> ("NewVal"=w341:bool)  [unwired: 1 in]
        n211 = case shown="False" w341 {
          tunnel: w340 -> [w350 _]
          tunnel: [w343 w361] -> w339
          tunnel: w338 -> [w342 w361]
          frame False {
            w357 = "Camera"
            w360 = FALSE ("Visible")
            n212 = local read "Camera Settings"() -> (w349:T2)
            n213 = Index Array(array=w350) -> (element=w353:cluster{string[]})  [unwired: 1 in]
            n214 = Unbundle(w349) -> ("Frame Rate"=w348:i32, "Compression"=w347:i32, "Size"=w351:u16)
            n215 = Unbundle(w353) -> (w352:string[])
            n216 = Index Array(array=w352, index=w351) -> (element=w346:string)
            n217 = call-poly <vilib>:"Write Key.vi"("section"=w357, "value"=w346, "key"="Size", "refnum"=w342) -> ("refnum out"=w359:T13)  [unwired: 2 in, 5 out]
            n218 = call-poly <vilib>:"Write Key.vi"("section"=w357, "value"=w348, "key"="FrameRate", "refnum"=w359) -> ("refnum out"=w358:T13)  [unwired: 1 in, 6 out]
            n219 = local write "DB Camera Config"(w360) -> ()
            n220 = property on="Camera Settings" class="Clust (strict)"("Visible"=w360) -> ()  [unwired: 2 in, 2 out]
            n221 = call-poly <vilib>:"Write Key.vi"("section"=w357, "value"=w347, "key"="Compression", "refnum"=w358) -> ("refnum out"=w344:T13)  [unwired: 1 in, 6 out]
            n222 = call <vilib>:"Close Config Data.vi"("refnum"=w344) -> ("file path"=w345:path)  [unwired: 2 in, 8 out]
            n223 = call <vilib>:"Open Config Data.vi"("configuration file path"=w345) -> ("refnum"=w343:T13)  [unwired: 8 in, 2 out]
          }
          frame True {
            n224 = property on="Camera Settings" class="Clust (strict)"("Visible"=TRUE) -> ()  [unwired: 2 in, 2 out]
          }
        }
      }
      event "Camera Settings": Value Change {
        n225 = event-data() -> ("NewVal"=w374:T2)  [unwired: 1 in]
        n226 = Index Array(array=w370) -> (element=w369:cluster{string[]})  [unwired: 1 in]
        n227 = Unbundle(w374) -> ("Frame Rate"=w365:i32, "Compression"=w364:i32, "Size"=w367:u16)
        n228 = Unbundle(w369) -> (w368:string[])
        n229 = Index Array(array=w368, index=w367) -> (element=w366:string)
        n230 = Format Into String(format string="%s   %dfps   %d%%", w366, w365, w364) -> (resulting string=w371:string)  [unwired: 2 in, 1 out]
        n231 = Build Array(w371) -> (w372:string[])
        n232 = property on="DB Camera Config" class="Bool (strict)"("Strings [4]"=w372) -> ()  [unwired: 2 in, 2 out]
      }
      event "Motor.Enable": Value Change {
        n233 = event-data() -> ("NewVal"=w380:bool)  [unwired: 1 in]
        n234 = Unbundle("Motor") -> ("Value"=w379:dbl)  [unwired: 1 out]
        n235 = Select(t=w379, s=w380, f=0.0) -> (s? t:f=w377:dbl)
        n236 = call <vilib>:"NT Write Number.vi"("Numeric"=w377, "Name"=w376) -> ()  [unwired: 9 in, 1 out]
      }
      event "Test Slider": Value Change {
        n237 = event-data() -> ("NewVal"=w383:dbl)  [unwired: 1 in]
        n238 = call <vilib>:"NT Write Number.vi"("Numeric"=w383, "Name"=w384) -> ()  [unwired: 9 in, 1 out]
      }
      event "On/Off": Value Change {
        n239 = event-data() -> ("NewVal"=w388:bool)  [unwired: 1 in]
        n240 = Boolean To (0,1)(Boolean=w388) -> (0, 1=w387:i16)
        n241 = call <vilib>:"NT Write Number.vi"("Numeric"=w387, "Name"=w386) -> ()  [unwired: 9 in, 1 out]
      }
      event "Rev/Fwd": Value Change {
        n242 = event-data() -> ("NewVal.Forward"=w396:bool, "NewVal.Reverse"=w395:bool)  [unwired: 1 in]
        n243 = Boolean To (0,1)(Boolean=w396) -> (0, 1=w392:i16)
        n244 = Boolean To (0,1)(Boolean=w395) -> (0, 1=w394:i16)
        n245 = Negate(x=w394) -> (-x=w393:i16)
        n246 = Add(x=w392, y=w393) -> (x+y=w391:i16)
        n247 = call <vilib>:"NT Write Number.vi"("Numeric"=w391, "Name"=w390) -> ()  [unwired: 9 in, 1 out]
      }
      event "Test Ring": Value Change {
        n248 = event-data() -> ("NewVal"=w400:u16)  [unwired: 1 in]
        n249 = property on="Test Ring" class="Ring (strict)"() -> ("Strings []"=w401:string[])  [unwired: 2 in, 2 out]
        n250 = Index Array(array=w401, index=w400) -> (element=w399:string)
        n251 = call <vilib>:"NT Write String.vi"("String"=w399, "Name"=w398) -> ()  [unwired: 9 in, 1 out]
      }
      event "Rec Mode": Value Change {
        # "Update globals for recording mode and path to read log from.\nClear when logging and let NetworkTables set path for vision to\nuse."
        n252 = event-data() -> ("NewVal"=w411:enum32{"Stop", "Record", "Playback"})  [unwired: 1 in]
        n253 = global write "WPI_DashboardLogging Global.vi" "Logging Filename"(path "") -> ()
        n254 = global write "WPI_DashboardLogging Global.vi" "Recording"(w411) -> ()
        n255 = case shown="\"Stop\", \"Record\"" w411 {
          tunnel: w410 -> [_ w413 w421]
          tunnel: [_ _ w420] -> w407
          tunnel: [_ _ w419] -> _
          tunnel: w405 -> [_ _ w417]
          tunnel: cluster{i32, i32} {-250, 170} -> [_ _ w416]
          tunnel: [_ _ T15 {"Image Size"=TRUE, "Image Type"=TRUE, "Pixel Value"=TRUE, "ROI Information"=TRUE, "Zoom Factor"=FALSE} ("Image Information Shown:All Elements")] -> w403
          tunnel: [_ _ TRUE ("Zoom Factor")] -> w402
          frame Default {
          }
          frame "Stop", "Record" {
            # "Place Window too"
            n256 = invoke class="VI" method="FP.Close"(reference=w413) -> (reference out=w412:refnum<vi>)  [unwired: 2 in, 2 out]
            n257 = invoke class="VI" method="Abort VI"(reference=w412) -> ()  [unwired: 2 in, 3 out]
          }
          frame "Playback" {
            n258 = call "Open Playback Panel.vi"("Offset"=w416, "DB VI Ref"=w417, "Playback in"=w421) -> ("Playback out"=w418:refnum<vi>)  [unwired: 8 in]
            n259 = register-events(w418) -> (reference out=w420:refnum<event-registration>, error out=w419:errorcluster)  [unwired: 2 in]
          }
        }
        n260 = property on="Camera Image" class="ImageControl"("Image Information Shown"=w403, "Image Information Visible"=w402) -> ()  [unwired: 2 in, 2 out]
        n261 = call <vilib>:"WPI_DashboardNT Log FieldName Cache.vi"("Operation"=enum16{"Lookup/Add", "Index", "Clear"}."Clear") -> ()  [unwired: 8 in, 3 out]
      }
      event Panel Close {
        w422 = enum32{"Stop", "Record", "Playback"}."Stop" ("Rec Mode")
        n262 = event-data() -> ()  [unwired: 1 in, 4 out]
        n263 = local write "Rec Mode"(w422) -> ()
        n264 = global write "WPI_DashboardLogging Global.vi" "Recording"(w422) -> ()
      }
      event Panel Close {
        # "Abort playback window and ourself"
        n265 = event-data() -> ()  [unwired: 1 in, 4 out]
        n266 = invoke class="VI" method="FP.Close"(reference=w427) -> (reference out=w426:refnum<vi>)  [unwired: 2 in, 2 out]
        n267 = invoke class="VI" method="Abort VI"(reference=w426) -> (error out=w425:errorcluster)  [unwired: 2 in, 2 out]
        n268 = invoke class="VI" method="Abort VI"(error in=w425) -> ()  [unwired: 2 in, 3 out]
      }
    }
  }
  n269 = property on="On/Off" class="Bool (strict)"("Visible"=w25) -> ()  [unwired: 2 in, 2 out]
  n270 = property on="Motor" class="Clust (strict)"("Visible"=w25) -> ()  [unwired: 2 in, 2 out]
  n271 = property on="Progress" class="Clust (strict)"("Visible"=w25) -> ()  [unwired: 2 in, 2 out]
  n272 = property on="Test Ring" class="Ring (strict)"("Visible"=w25) -> ()  [unwired: 2 in, 2 out]
  n273 = property on="Rev/Fwd" class="Clust (strict)"("Visible"=w25) -> ()  [unwired: 2 in, 2 out]
  n274 = local write "DB Camera Config"(w25) -> ()
  n275 = property on="Camera Settings" class="Clust (strict)"("Visible"=w25) -> ()  [unwired: 2 in, 2 out]
  n276 = global write "WPI_DashboardLogging Global.vi" "Recording"(w8) -> ()
  n277 = local write "Rec Mode"(w8) -> ()
